vi "sub_get_Device_ID.vi"(8 "error in (no error)":errorcluster, 11 "daq.io type in":T1={"daq.io ref"=refnum, "daq.io API Base"="http://dashboard.daq.io/api/v1", "Device Type Key"="", "Device Key"="", "Account ID"="", "online"=FALSE}) -> (0 "error out":errorcluster, 2 "Device ID":string, 3 "daq.io type out":T1={"daq.io ref"=refnum, "daq.io API Base"="http://dashboard.daq.io/api/v1", "Device Type Key"="", "Device Key"="", "Account ID"="", "online"=FALSE})   [LabVIEW 2013, in "daqio minimal.lvlib"]
uses:
  daqio minimal.lvlib
  <vilib>/httpClient/ClientHandle.ctl
  <vilib>/httpClient/LabVIEWHTTPClient.lvlib
  _typedefs/daqio-Type.ctl
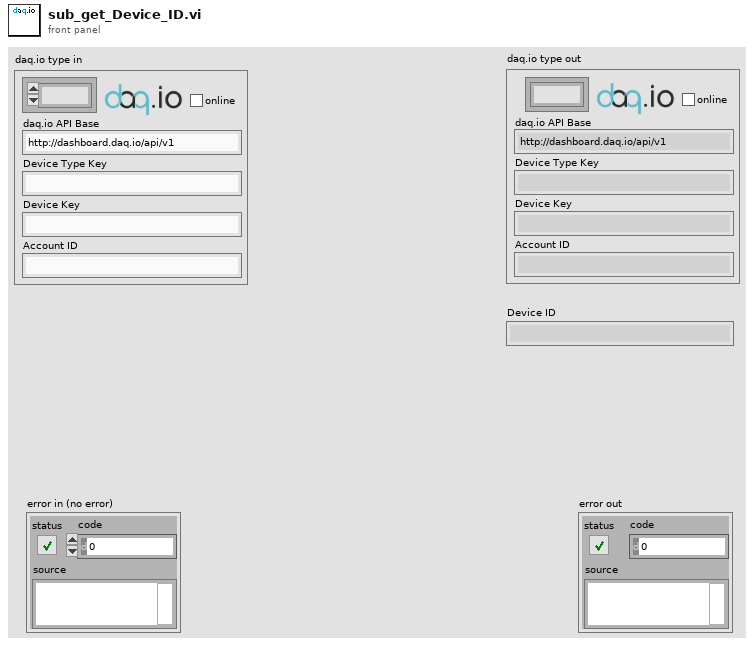
[diagram p1: front panel]
types:
  T1 = typedef "daqio minimal.lvlib/daqio-Type.ctl" = cluster{"daq.io ref":T2, "daq.io API Base":string, "Device Type Key":string, "Device Key":string, "Account ID":string, "online":bool}
  T2 = typedef "LabVIEWHTTPClient.lvlib/ClientHandle.ctl" = refnum<k1>
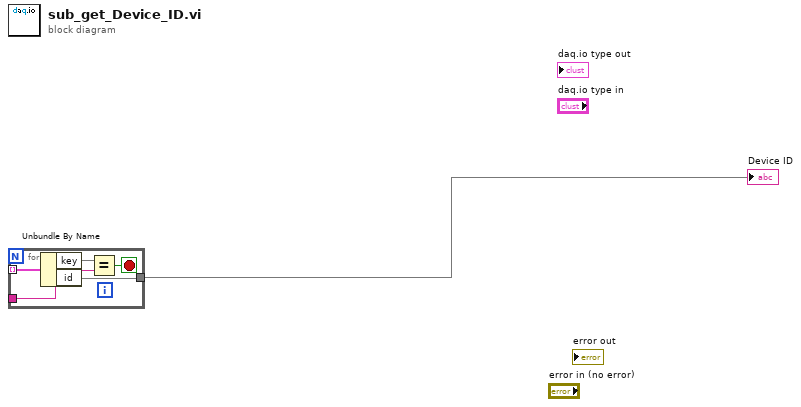
[diagram p0: block diagram]
diagram:
  n1 = for {
    tunnel: [w7] -> w1 mode=indexing
    tunnel: _ -> [w4]
    tunnel: [w3] -> w2
    stop <- w5 stop-if-true
    n2 = Unbundle By Name(w7) -> ("key"=w6, "id"=w3)
    n3 = Equal?(x=w6, y=w4) -> (x = y?=w5:bool)
  }
  "Device ID" <- w2
